vi "Append VI Hierarchy to Report (refnum).vi"(0 "report in":refnum<class "NI_report.lvclass">, 2 "image format (jpeg)":enum32{"PNG", "JPEG", "GIF"}(ring)=enum."JPEG", 5 "VI":refnum<vi>, 7 "alignment (default)":T2, 11 "error in (no error)":errorcluster, 12 "MS Office parameters":T1) -> (4 "report out":refnum<class "NI_report.lvclass">, 6 "VI out":refnum<vi>, 8 "start out (Word)":i32, 10 "end out (Word)":i32, 15 "error out":errorcluster)   [LabVIEW 2020, in "NI_ReportGenerationCore.lvlib"]
doc: "Appends the hierarchy of the VI you specify in <B>VI</B> to a report. Wire data to the <B>VI</B> input to determine the polymorphic instance to use or manually select the instance."
uses:
  <vilib>/Utility/NIReport.llb/NI_ReportGenerationCore.lvlib
  <vilib>/Utility/NIReport.llb/NI_report.lvclass
  <vilib>/Utility/NIReport.llb/HTML Report Image Alignment.ctl
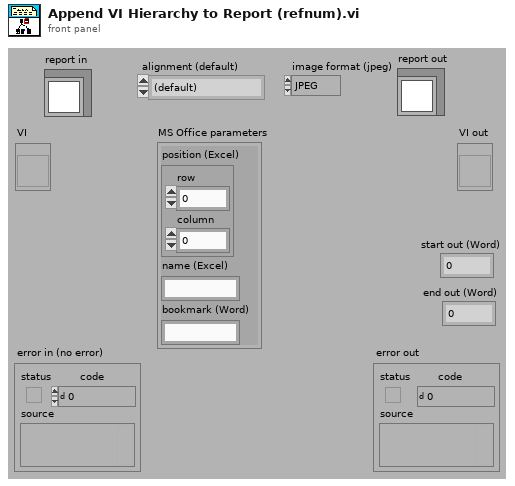
[diagram p1: front panel]
types:
  T1 = cluster{"position (Excel)":cluster{"row":i32, "column":i32}, "name (Excel)":string, "bookmark (Word)":string}
  T2 = typedef "NI_ReportGenerationCore.lvlib/HTML Report Image Alignment.ctl" = enum16{"(default)", "LEFT", "RIGHT", "TOP", "TEXTTOP", "MIDDLE", "ABSMIDDLE", "BASELINE", "BOTTOM", "ABSBOTTOM"}
  T3 = enum32{"invalid app kind", "Development System", "Run Time System", "Student Edition", "Embedded LabVIEW", "Evaluation", "Custom"}
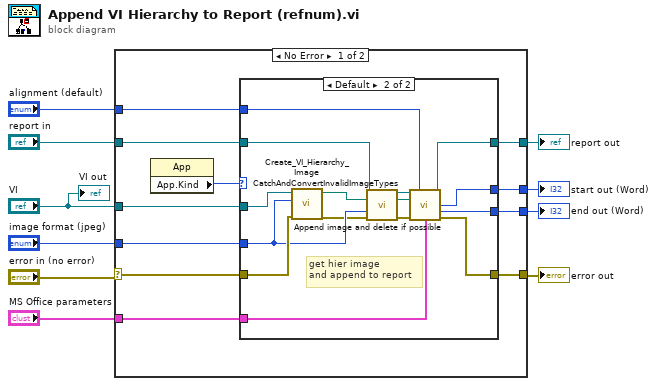
[diagram p0: block diagram]
diagram:
  n1 = case shown="No Error" "error in (no error)" {
    selector: "error in (no error)" -> [w21 w40]
    tunnel: [w19 w40] -> w9
    tunnel: "report in" -> [w13 w39]
    tunnel: "VI" -> [w20 _]
    tunnel: "image format (jpeg)" -> [w18 _]
    tunnel: "alignment (default)" -> [w17 _]
    tunnel: "MS Office parameters" -> [w16 _]
    tunnel: [w15 _] -> w3
    tunnel: [w14 _] -> w2
    tunnel: [w12 w39] -> w1
    frame No Error {
      n2 = property class="App"() -> ("App.Kind"=w11:T3)  [unwired: 2 in, 2 out]
      n3 = case shown="Default" w11 {
        tunnel: w21 -> [w22 w38]
        tunnel: w20 -> [_ w37]
        tunnel: [w22 w36] -> w19
        tunnel: w18 -> [_ w32]
        tunnel: w17 -> [_ w30]
        tunnel: w16 -> [_ w29]
        tunnel: [_ w28] -> w15
        tunnel: [_ w27] -> w14
        tunnel: w13 -> [w23 w25]
        tunnel: [w23 w24] -> w12
        frame "Run Time System" {
          # "Do not try to append\nif running in an\nexecutable"
        }
        frame Default {
          # "get hier image\nand append to report"
          n4 = call <vilib>:"Create_VI_Hierarchy_Image.vi"("error in (no error)"=w38, "Image Format (jpeg)"=w32, "VI"=w37) -> ("error out"=w31:errorcluster, "Path to image"=w26:path)  [unwired: 7 in]
          n5 = call-dynamic "CatchAndConvertInvalidImageTypes.vi"("report in"=w25, "path to image"=w26, "image format (jpeg)"=w32, "error in (no error)"=w31) -> ("report out"=w33:refnum<class "NI_report.lvclass">, "path to image out"=w34:path, "error out"=w35:errorcluster)  [unwired: 9 in]
          n6 = call-dynamic "Append image and delete if possible.vi"("report in"=w33, "alignment (default)"=w30, "path to image"=w34, "error in (no error)"=w35, "MS Office parameters"=w29) -> ("report out"=w24:refnum<class "NI_report.lvclass">, "start out Word)"=w28:i32, "end out Word)"=w27:i32, "error out"=w36:errorcluster)  [unwired: 7 in]
        }
      }
    }
    frame Error {
    }
  }
  "error out" <- w9
  "report out" <- w1
  "start out (Word)" <- w3
  "end out (Word)" <- w2
  "VI out" <- "VI"
